vi "Main_Calculations.vi"(0 "Controls":T2) -> (4 "Indicators":T1)   [LabVIEW 2018]
doc: "This VI contains the following:\n\nSub VI:\nGravity_Calculation;\nCurrent_Linear_Speed;\nLinear_Distance;\nCurrent_Rotary_Speed;\nNumber_Of_Rotations.\n\nControls:\nArray prev;\nLinear Distance prev;\nAxle Radius;\nNumber of Rotations prev;\nNo. of Slits;\nEncoder Count;\nCurrent Linear Speed Prev.\n\nIndicators:\nChange in Linear Distance;\nArray;\nCurent Linear Speed;\nAcceleration due to Gravity;\nNumber of Rotations;\nCurrent Rotary Speed;\nLinear Distance."
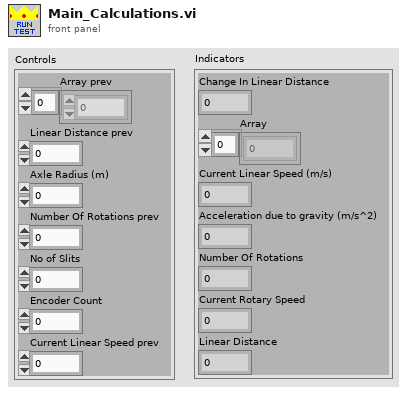
[diagram p1: front panel]
types:
  T1 = cluster{"Change In Linear Distance":dbl, "Array":dbl[], "Current Linear Speed (m/s)":dbl, "Acceleration due to gravity (m/s^2)":dbl, "Number Of Rotations":dbl, "Current Rotary Speed":dbl, "Linear Distance":dbl}
  T2 = cluster{"Array prev":dbl[], "Linear Distance prev":dbl, "Axle Radius (m)":dbl, "Number Of Rotations prev":dbl, "No of Slits":dbl, "Encoder Count":dbl, "Current Linear Speed prev":dbl}
  T3 = cluster{"Change In Linear Distance":dbl, "Array ":dbl[], "Current Linear Speed":dbl, "Acceleration due to gravity":dbl, "Number Of Rotations":dbl, "Current Rotary Speed":dbl, "Linear Distance":dbl}
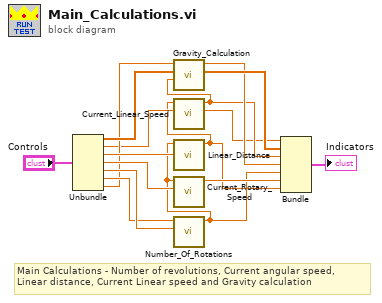
[diagram p0: block diagram]
diagram:
  # "Main Calculations - Number of revolutions, Current angular speed,\nLinear distance, Current Linear speed and Gravity calculation"
  n1 = Unbundle("Controls") -> ("Array prev"=w15:dbl[], "Linear Distance prev"=w9:dbl, "Axle Radius (m)"=w12:dbl, "Number Of Rotations prev"=w11:dbl, "No of Slits"=w14:dbl, "Encoder Count"=w13:dbl, "Current Linear Speed prev"=w10:dbl)
  n2 = call "Number_Of_Rotations.vi"("No of Slits"=w14, "Encoder Count"=w13) -> ("Number Of Rotations"=w5:dbl)  [unwired: 9 in]
  n3 = call "Linear_Distance.vi"("Axle Radius"=w12, "Number Of Rotations"=w5) -> ("Linear Distance"=w3:dbl)  [unwired: 9 in]
  n4 = call "Current_Linear_Speed.vi"("Linear Distance prev"=w9, "Linear Distance"=w3) -> ("Change In Linear Distance"=w1:dbl, "Current Linear Speed"=w2:dbl)  [unwired: 8 in]
  n5 = call "Gravity_Calculation.vi"("Current Linear Speed"=w2, "Array prev"=w15, "Current Linear Speed prev"=w10) -> ("Array"=w8:dbl[], "Acceleration due to gravity"=w4:dbl)  [unwired: 6 in]
  n6 = call "Current_Rotary_Speed.vi"("Number Of Rotations prev"=w11, "Number Of Rotations"=w5) -> ("Current Rotary Speed"=w6:dbl)  [unwired: 9 in]
  n7 = Bundle("Change In Linear Distance"=w1, "Array"=w8, "Current Linear Speed"=w2, "Acceleration due to gravity"=w4, "Number Of Rotations"=w5, "Current Rotary Speed"=w6, "Linear Distance"=w3) -> (→"Indicators":T3)  [unwired: 1 in]
